vi "(SubVI)I2C_Log_Sequential.vi"(5 "Data Size":T1, 7 "R/W":T2, 8 "error in (no error)":errorcluster caption="에러 입력(에러 없음)", 9 "Data Array":i16[](array[numeric]), 10 "Start Address":u16, 11 "Log Ref":refnum<vi>) -> (0 "error out":errorcluster caption="에러 출력", 3 "Log":string)   [LabVIEW 2020]
uses:
  Controls/(Ctrl)I2C_RW.ctl
  Controls/(Ctrl)I2C_Data Size.ctl
panel:
  # "(SubVI)I2C_Log_Sequential.vi By hspark\n\nDescription : I2C Sequential Read/Write 동작에 대해 (SubVI)I2C_Log.vi를 사용할 수 있도록 작성된 VI\n\nInput : \n1. Log Ref : 업데이트할 Log 문자열 인디케이터의 참조. 입력하지 않는 경우 Log 문자열만 출력하고, 인디케이터 업데이트는 무시됨\n2. Start Address : Sequential Read/Write 동작의 Start Address\n3. Data : Sequential Read/Wirte 동작의 Data\n4. R/W : Read/Write 구분\n5. Data Size : 생성할 Log의 비트 크기\n\nOutput : \n1. Log : 생성된 Log 문자열 출력\n\nLabVIEW Version : 2020 SP1 이상\n\nNote : 에러 발생 시 에러 종류를 Log로 출력함. \n\nUpdate : 2021.10.06"
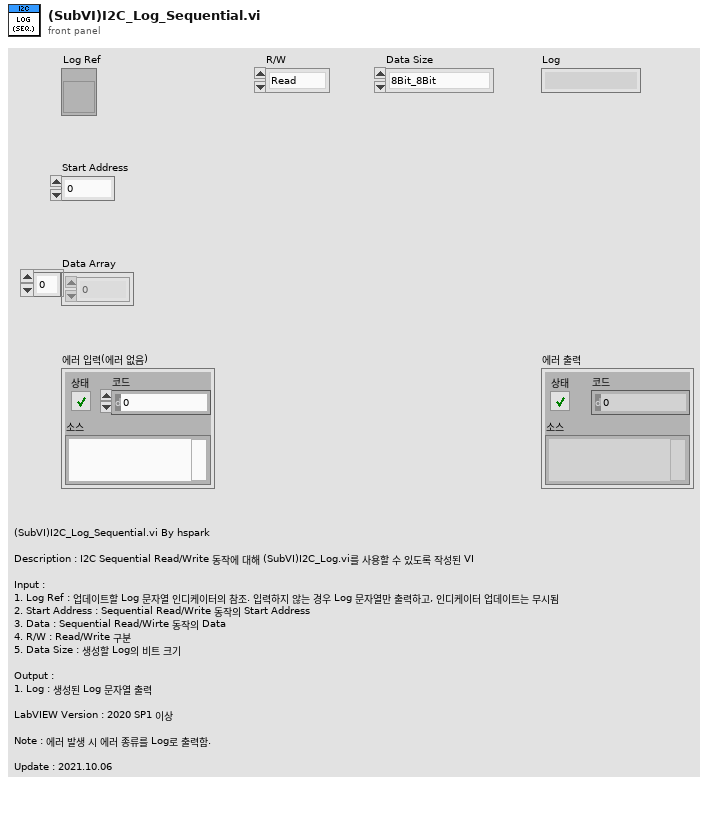
[diagram p1: front panel]
types:
  T1 = typedef "(Ctrl)I2C_Data Size.ctl" = enum16{"8Bit_8Bit", "16Bit_16Bit", "16Bit_8Bit"}
  T2 = typedef "(Ctrl)I2C_RW.ctl" = enum16{"Read", "Write"}
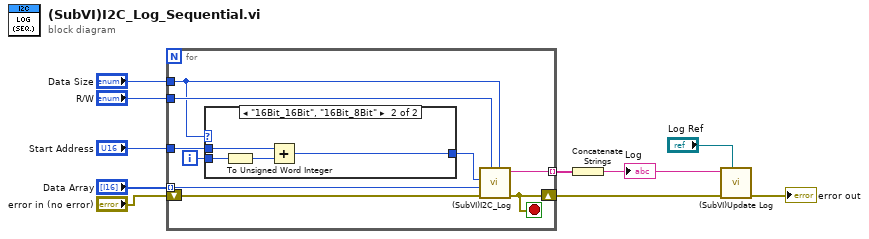
[diagram p0: block diagram]
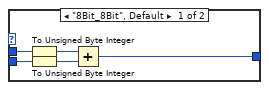
[diagram p2: hidden frame]
diagram:
  n1 = for {
    tunnel: "Start Address" -> [w14]
    tunnel: "Data Array" -> [w18] mode=indexing
    shift-right: [w11] -> w10
    shift-left: "error in (no error)" -> [w19]
    tunnel: [w17] -> w9 mode=indexing
    tunnel: "R/W" -> [w16]
    tunnel: "Data Size" -> [w15]
    i -> [w13]
    stop <- w11 stop-if-true
    n2 = case shown="\"16Bit_16Bit\", \"16Bit_8Bit\"" w15 {
      tunnel: w14 -> [w24 w25]
      tunnel: w13 -> [w23 w28]
      tunnel: [w20 w26] -> w12
      frame "8Bit_8Bit", Default {
        n3 = To Unsigned Byte Integer(number=w24) -> (unsigned 8bit integer=w22:u8)
        n4 = To Unsigned Byte Integer(number=w23) -> (unsigned 8bit integer=w21:u8)
        n5 = Add(x=w22, y=w21) -> (x+y=w20:u8)
      }
      frame "16Bit_16Bit", "16Bit_8Bit" {
        n6 = To Unsigned Word Integer(number=w28) -> (unsigned 16bit integer=w27:u16)
        n7 = Add(x=w25, y=w27) -> (x+y=w26:u16)
      }
    }
    n8 = call "(SubVI)I2C_Log.vi"("Data Size"=w15, "R/W"=w16, "error in (no error)"=w19, "Data"=w18, "Address"=w12) -> ("error out"=w11:errorcluster, "Log"=w17:string)  [unwired: 5 in]
  }
  n9 = Concatenate Strings(w9) -> (w8:string)
  "Log" <- w8
  n10 = call "(SubVI)Update Log.vi"("Log Ref"="Log Ref", "error in (no error)"=w10, "Log"=w8) -> ("error out"=→"error out":errorcluster)  [unwired: 7 in, 1 out]
